vi "uMsg Create.vi"(4 "Reply Payload":refnum<class "uData.lvclass">, 5 "Reply CMD (re:<cmd>)":string, 6 "Timestamp (NULL)":u32, 7 "Reply Transport":refnum<class "uTransport.lvclass">, 8 "error in (no error)":errorcluster, 10 "Payload":refnum<class "uData.lvclass">, 11 "CMD":string) -> (0 "error out":errorcluster, 3 "uMsg out":refnum<class "uMsg.lvclass">)   [LabVIEW 2023, in "uLib.lvlib" / "uMsg.lvclass"]
doc: "This method executes regardless of the error state."
uses:
  uMsg.lvclass
  uData/uData/uData.lvclass
  uTransport/uTransport/uTransport.lvclass
  uMsg.lvclass/uMsg.ctl
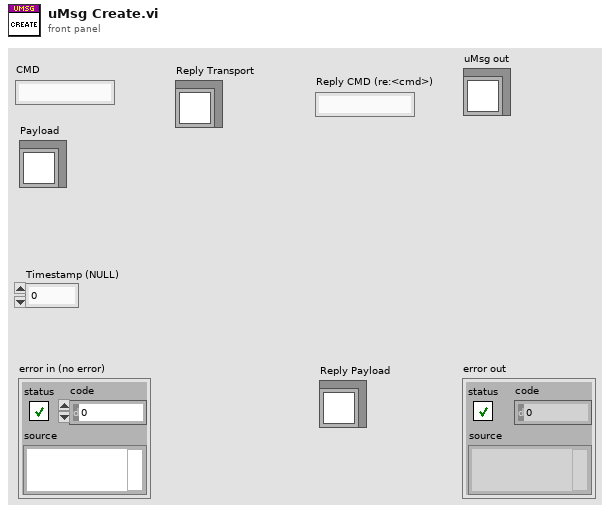
[diagram p1: front panel]
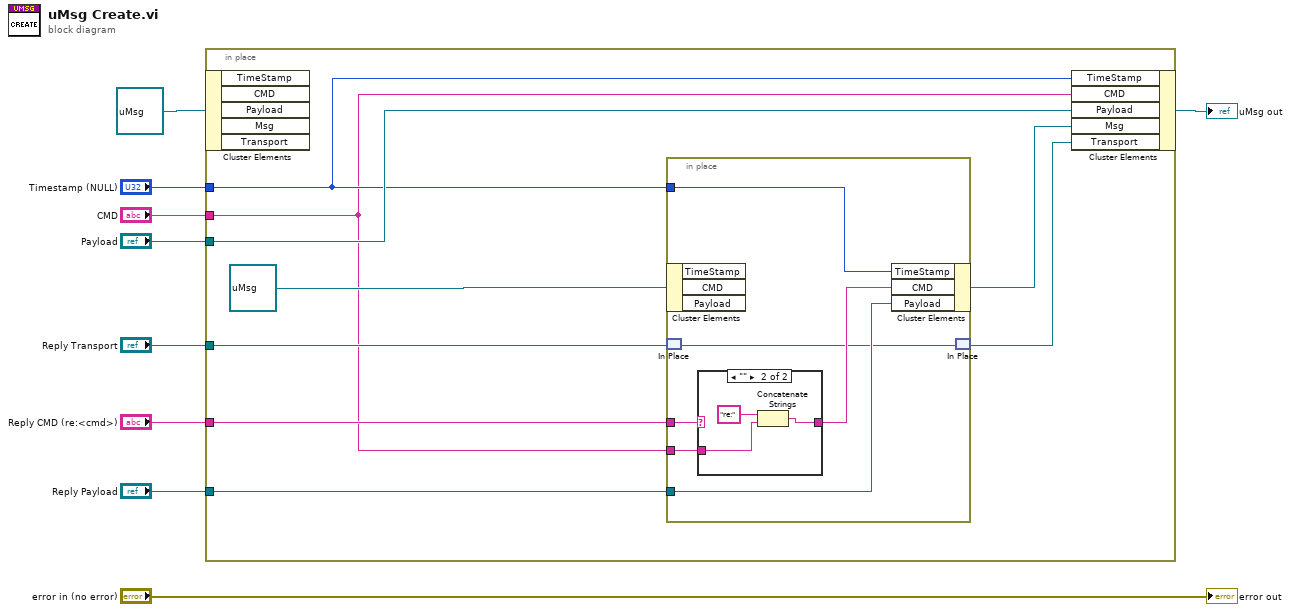
[diagram p0: block diagram]
diagram:
  n1 = in-place {
    in-place-border: "CMD" -> [w10]
    in-place-border: "Payload" -> [w18]
    in-place-border: "Timestamp (NULL)" -> [w17]
    in-place-border: "Reply Transport" -> [w12]
    in-place-border: "Reply Payload" -> [w16]
    in-place-border: "Reply CMD (re:<cmd>)" -> [w15]
    n2 = in-place-cluster #1(refnum<class "uMsg.lvclass"> refnum ("uMsg in")) -> ()  [unwired: 5 out]
    n3 = in-place {
      in-place-border: w17 -> [w24]
      in-place-border: w16 -> [w23]
      in-place-border: w15 -> [w22]
      in-place-border: w10 -> [w19]
      n4 = in-place-cluster #2(refnum<class "uMsg.lvclass"> refnum ("uMsg in")) -> ()  [unwired: 3 out]
      n5 = in-place-match #3(w12) -> (w20:refnum<class "uTransport.lvclass">)
      n6 = case shown="\"\"" w22 {
        selector: w22 -> [w25 _]
        tunnel: [w25 w28] -> w21
        tunnel: w19 -> [_ w26]
        frame Default {
        }
        frame "" {
          n7 = Concatenate Strings("re:" ("string"), w26) -> (w28:string)
        }
      }
      n8 = in-place-cluster #2("TimeStamp"=w24, "CMD"=w21, "Payload"=w23) -> (w14:refnum<class "uMsg.lvclass">)
      n9 = in-place-match #3(w20) -> (w11:refnum<class "uTransport.lvclass">)
    }
    n10 = in-place-cluster #1("TimeStamp"=w17, "CMD"=w10, "Payload"=w18, "Msg"=w14, "Transport"=w11) -> (→"uMsg out":refnum<class "uMsg.lvclass">)
  }
  "error out" <- "error in (no error)"
